vi "VI - Interactive or SubVI.vi"() -> (1 "Mode":T1)   [LabVIEW 2013]
uses:
  Controls/Enum - InteractiveMode-SubVIMode.ctl
panel:
  in  "Including itself":bool=TRUE
  out "call chain":string[](array[string])=["Untitled 2"]
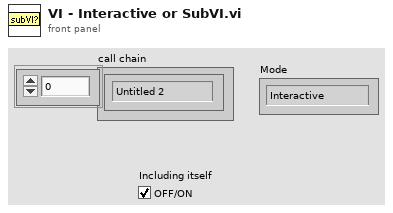
[diagram p1: front panel]
types:
  T1 = typedef "Enum - InteractiveMode-SubVIMode.ctl" = enum16{"Interactive", "subVI Mode"}
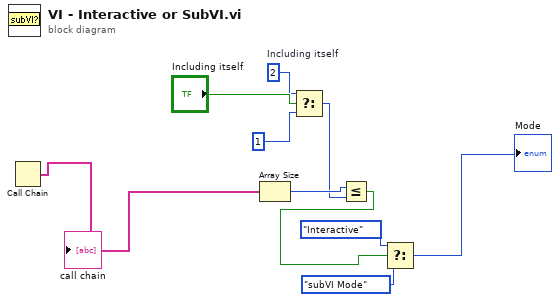
[diagram p0: block diagram]
diagram:
  w3 = 2  # Including itself
  n1 = Call Chain() -> (call chain=w9:string[])
  "call chain" <- w9
  n2 = Array Size(array=w9) -> (size(s)=w5:i32)
  n3 = Select(t=w3, s="Including itself", f=1) -> (s? t:f=w1:i32)
  n4 = Less Or Equal?(x=w5, y=w1) -> (x <= y?=w6:bool)
  n5 = Select(t=Enum_-_InteractiveMode-SubVIMode."Interactive", s=w6, f=Enum_-_InteractiveMode-SubVIMode."subVI Mode") -> (s? t:f=→"Mode":T1)
